vi "Constants.vi"() -> ()   [LabVIEW 2019, in "Telemetry Shared.lvlib"]
doc: "Use this Global VI to access the GUIDs assigned to the page resources of the Custom Device."
uses:
  Telemetry Shared.lvlib
panel:
  in  "Tab Control":enum32{"GUIDs", "Constants", "Properties"}(tab)
  in  "File Page GUID":string="665e130f-6b1d-4741-ab4b-127a5bcde637"
  in  "Telemetry GUID":string="93888e30-d6eb-4f06-90c8-66464dbab1ea"
  in  "Log File Path":string="Log File Path"
  in  "Overwrite File If Exists?":string="Overwrite File If Exists?"
  in  "Compiled.Settings":string="Compiled.Settings"
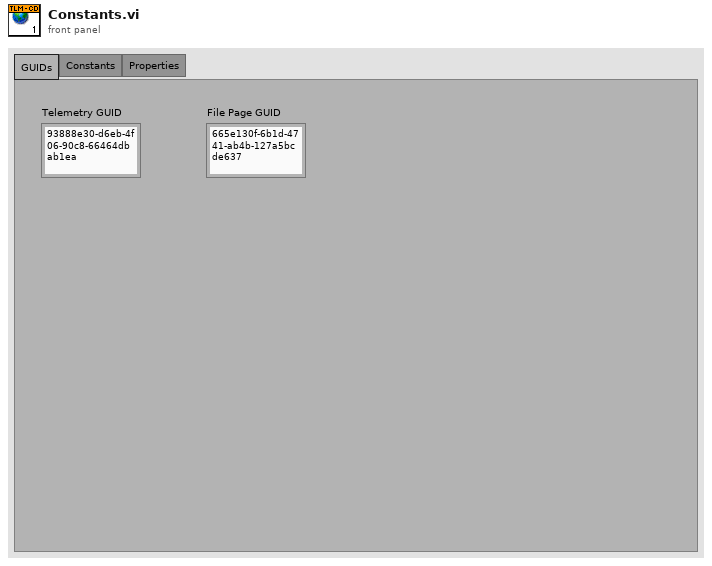
[diagram p1: front panel]
diagram:
